vi "Configure.vi"(8 "error in (no error)":errorcluster, 11 "Mag Lab Measure Interface in":refnum<class "Mag Lab Measure UI.lvclass">) -> (0 "error out":errorcluster, 3 "Mag Lab Measure Interface out":refnum<class "Mag Lab Measure UI.lvclass">)   [LabVIEW 2015, in "Mag Lab Measure UI.lvclass"]
uses:
  Mag Lab Measure UI.lvclass
  Mag Lab Measure UI.lvclass/Mag Lab Measure UI.ctl
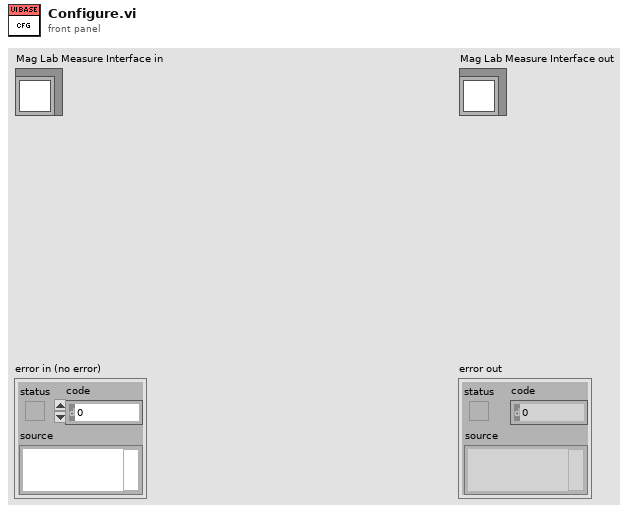
[diagram p1: front panel]
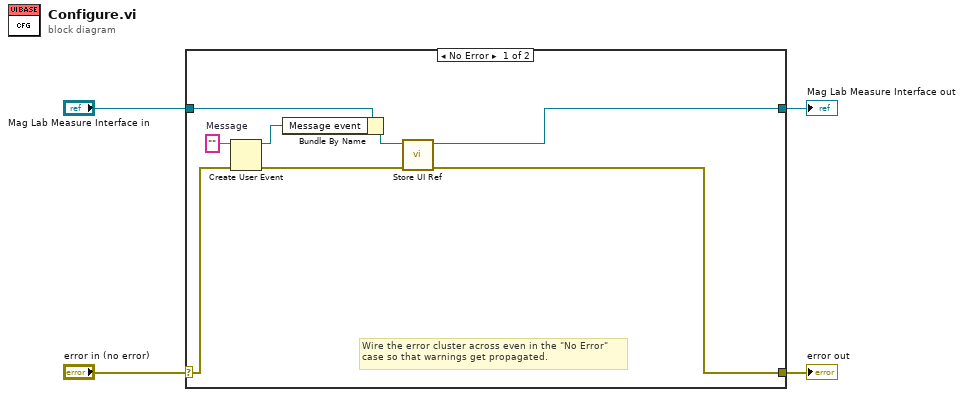
[diagram p0: block diagram]
diagram:
  n1 = case shown="No Error" "error in (no error)" {
    selector: "error in (no error)" -> [w10 w14]
    tunnel: [w6 w14] -> w3
    tunnel: [w5 w13] -> w1
    tunnel: "Mag Lab Measure Interface in" -> [w12 w13]
    frame No Error {
      w11 = ""  # Message
      # "Wire the error cluster across even in the \"No Error\"\ncase so that warnings get propagated."
      n2 = Create User Event(user event datatype=w11, error in=w10) -> (user event=w7:refnum<user-event>, error out=w9:errorcluster)
      n3 = Bundle By Name(cluster=w12, "Message event"=w7) -> (w8:refnum<class "Mag Lab Measure UI.lvclass">)
      n4 = call "Store UI Ref.vi"("error in (no error)"=w9, "Mag Lab Measure Interface in"=w8) -> ("error out"=w6:errorcluster, "Mag Lab Measure Interface out"=w5:refnum<class "Mag Lab Measure UI.lvclass">)  [unwired: 8 in]
    }
    frame Error {
    }
  }
  "error out" <- w3
  "Mag Lab Measure Interface out" <- w1
